vi "VIremotePaletteVIs.vi"(11 "Strings [] Demo VIs":string[](array[string])) -> (1 "Strings [] Controls":string[](array[string]), 5 "Array":T5(array[cluster]) {"Palette Type" items=["Functions"=-1, "Controls"=-2]; "View Format" items=["Icons", "Text", "Icons and Text"]})   [LabVIEW 2011]
uses:
  <vilib>/Palette API/Palette Menu/Public Type Define/View Format.ctl
  <vilib>/Palette API/Palette Menu/Public Type Define/Palette type.ctl
  VIremote.llb/VIremoteEvent.ctl
  VIremote.llb/VIremoteBarButton.ctl
  <vilib>/Palette API/Palette Menu/Palette Menu.lvlib
panel:
  in  "Bar Button":T1
  in  "VIremoteEvent":T2
  in  "New":i32(listbox)
  in  "1.Connection":i32(listbox)
  in  "VIremote":i32(listbox) caption="Controls"
  in  "2.Misc.":i32(listbox)
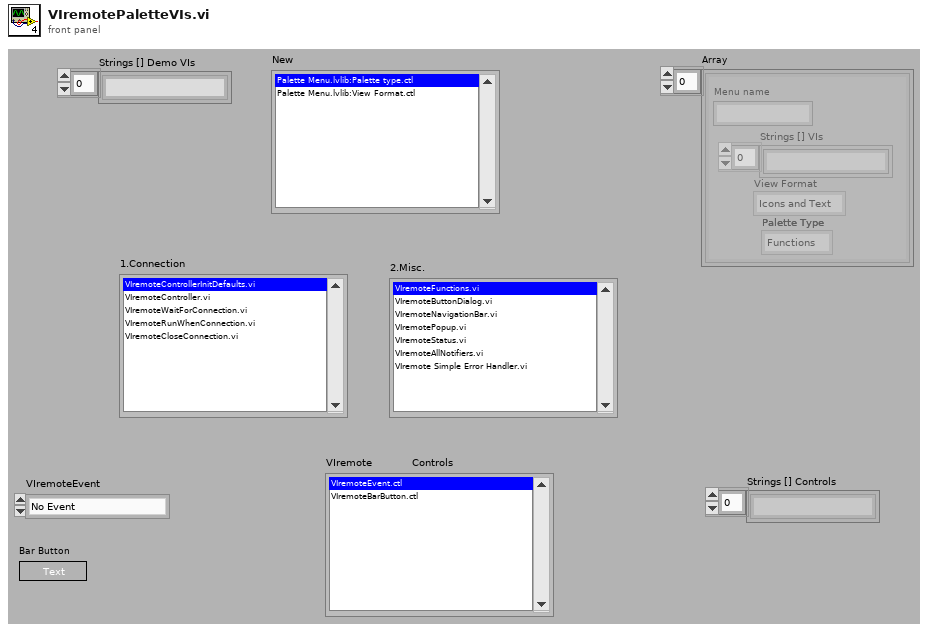
[diagram p1: front panel]
types:
  T1 = typedef "VIremoteBarButton.ctl" = bool
  T2 = typedef "VIremoteEvent.ctl" = enum16{"No Event", "Connection Closed", "Navigate Back", "Enter Background", "Enter Foreground", "Portrait", "Portrait Upside Down", "Landscape Left", "Landscape Right"}
  T3 = typedef "Palette Menu.lvlib/View Format.ctl" = u16
  T4 = typedef "Palette Menu.lvlib/Palette type.ctl" = i32
  T5 = cluster{"Menu name":string, "Strings [] VIs":string[], "View Format":T3, "Palette Type":T4}[]
  T6 = enum8{"Only include commented out diagrams if diagram already loaded", "Never include commented out diagrams", "Always include commented out diagrams"}
  T7 = cluster{"Label.Text":string, "Item Names":string[], "view format":T3, "palette type":T4}
  T8 = cluster{"Label.Text":string, "Item Names":string[], "view format":T3, "palette type":T4}[]
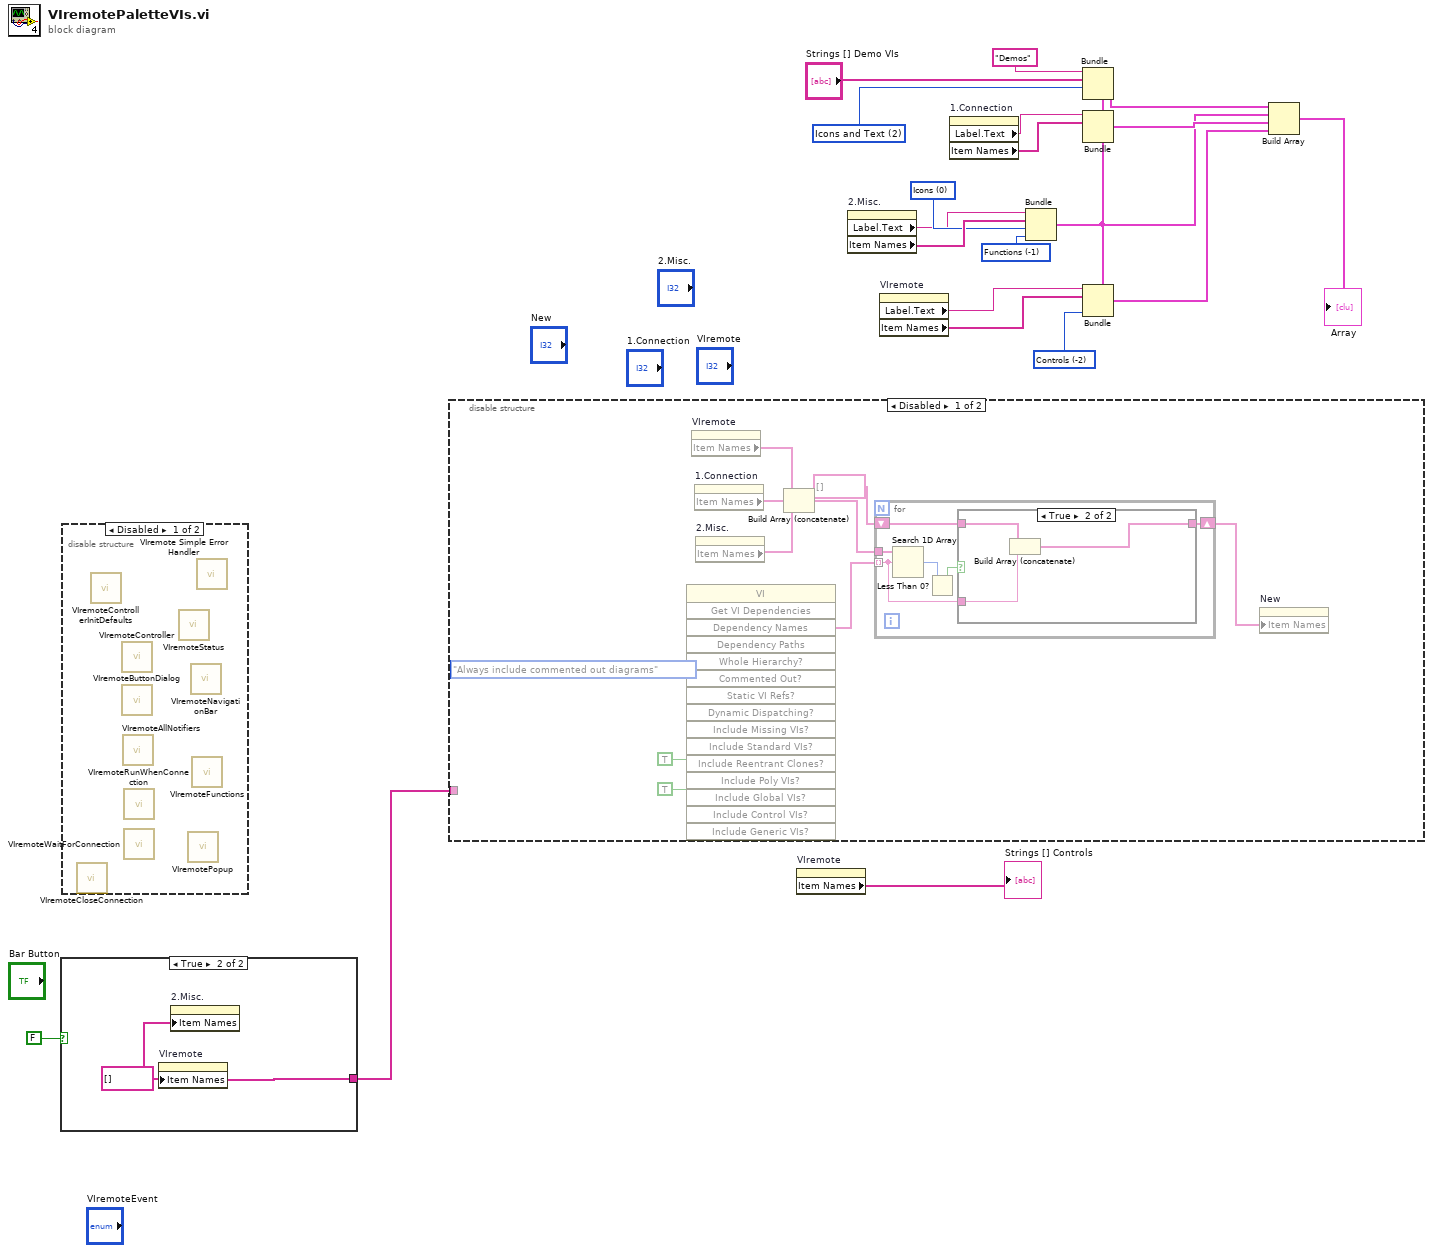
[diagram p0: block diagram]
diagram:
  w2 = T4 -2 items=["Functions"=-1, "Controls"=-2] ("palette type")
  w6 = T4 -1 items=["Functions"=-1, "Controls"=-2] ("palette type")
  w9 = T3 0 items=["Icons", "Text", "Icons and Text"] ("view format")
  w10 = T3 2 items=["Icons", "Text", "Icons and Text"] ("view format")
  n1 = case shown="True" FALSE {
    tunnel: [_ w21] -> w18
    frame False {
    }
    frame True {
      w21 = string[] [] ("Item Names")
      n2 = property on="VIremote" class="LstBox (strict)"("Item Names"=w21) -> ()  [unwired: 2 in, 2 out]
      n3 = property on="2.Misc." class="LstBox (strict)"("Item Names"=w21) -> ()  [unwired: 2 in, 2 out]
    }
  }
  n4 = disable-structure shown="Disabled" {
    frame Disabled {
      n5 = call "VIremoteCloseConnection.vi"() -> ()  [unwired: 11 in, 1 out]
      n6 = call "VIremoteControllerInitDefaults.vi"() -> ()  [unwired: 11 in, 1 out]
      n7 = call "VIremoteController.vi"() -> ()  [unwired: 12 in]
      n8 = call "VIremoteButtonDialog.vi"() -> ()  [unwired: 10 in, 2 out]
      n9 = call "VIremoteAllNotifiers.vi"() -> ()  [unwired: 10 in, 2 out]
      n10 = call "VIremoteRunWhenConnection.vi"() -> ()  [unwired: 11 in, 1 out]
      n11 = call "VIremoteWaitForConnection.vi"() -> ()  [unwired: 11 in, 1 out]
      n12 = call "VIremoteStatus.vi"() -> ()  [unwired: 3 in, 9 out]
      n13 = call "VIremotePopup.vi"() -> ()  [unwired: 10 in, 2 out]
      n14 = call "VIremoteNavigationBar.vi"() -> ()  [unwired: 11 in, 1 out]
      n15 = call "VIremoteFunctions.vi"() -> ()  [unwired: 11 in, 1 out]
      n16 = call "VIremote Simple Error Handler.vi"() -> ()  [unwired: 5 in, 5 out]
    }
    frame Enabled {
    }
  }
  n17 = disable-structure shown="Disabled" {
    disable-tunnel: w18 -> [_ _]
    frame Disabled {
      n18 = invoke class="VI" method="Get VI Dependencies"("Commented Out?"=T6."Always include commented out diagrams" ("Commented Out Diagrams?"), "Include Poly VIs?"=TRUE, "Include Control VIs?"=TRUE) -> ("Dependency Names"=w30:string[])  [unwired: 13 in, 15 out]
      n19 = property on="VIremote" class="LstBox (strict)"() -> ("Item Names"=w22:string[])  [unwired: 2 in, 2 out]
      n20 = property on="1.Connection" class="LstBox (strict)"() -> ("Item Names"=w27:string[])  [unwired: 2 in, 2 out]
      n21 = property on="2.Misc." class="LstBox (strict)"() -> ("Item Names"=w26:string[])  [unwired: 2 in, 2 out]
      n22 = Build Array (concatenate)(w22, w27, w26) -> (w25:string[])
      n23 = for {
        tunnel: w25 -> [w37]
        tunnel: w30 -> [w33] mode=indexing
        shift-right: [w32] -> w24
        shift-left: string[] [] -> [w34]
        n24 = Search 1D Array(1D array=w37, element=w33) -> (index of element=w36:i32)  [unwired: 1 in]
        n25 = Less Than 0?(x=w36) -> (x < 0?=w35:bool)
        n26 = case shown="True" w35 {
          tunnel: w34 -> [w38 w41]
          tunnel: w33 -> [_ w40]
          tunnel: [w38 w39] -> w32
          frame False {
          }
          frame True {
            n27 = Build Array (concatenate)(w41, w40) -> (w39:string[])
          }
        }
      }
      n28 = property on="New" class="LstBox (strict)"("Item Names"=w24) -> ()  [unwired: 2 in, 2 out]
    }
    frame Enabled {
    }
  }
  n29 = property on="VIremote" class="LstBox (strict)"() -> ("Item Names"=→"Strings [] Controls":string[])  [unwired: 2 in, 2 out]
  n30 = property on="2.Misc." class="LstBox (strict)"() -> ("Label.Text"=w7:string, "Item Names"=w14:string[])  [unwired: 2 in, 2 out]
  n31 = property on="VIremote" class="LstBox (strict)"() -> ("Label.Text"=w4:string, "Item Names"=w3:string[])  [unwired: 2 in, 2 out]
  n32 = property on="1.Connection" class="LstBox (strict)"() -> ("Label.Text"=w8:string, "Item Names"=w15:string[])  [unwired: 2 in, 2 out]
  n33 = Bundle("Label.Text"=w7, "Item Names"=w14, "view format"=w9, "palette type"=w6) -> (w5:T7)  [unwired: 1 out]
  n34 = Bundle(cluster=w5, "Label.Text"="Demos", "Item Names"="Strings [] Demo VIs", "view format"=w10) -> (w12:T7)  [unwired: 1 out]
  n35 = Bundle(cluster=w5, "Label.Text"=w8, "Item Names"=w15) -> (w13:T7)  [unwired: 2 out]
  n36 = Bundle(cluster=w5, "Label.Text"=w4, "Item Names"=w3, "palette type"=w2) -> (w1:T7)  [unwired: 1 out]
  n37 = Build Array(w12, w5, w13, w1) -> (→"Array":T8)
